vi "Delimited path to array.vi"(8 "error in (no error)":errorcluster, 10 "Node Path Delimited (parent, child)":string, 11 "Tree Map Handle In":T1) -> (0 "error out":errorcluster, 2 "Node Path (parent, child)":string[](array[string]), 3 "Tree Map Handle out":T1)   [LabVIEW 2020, in "Blue Tree Map OpenSource.lvlib"]
doc: "This functions converts a delimited string to a string array.\n\nThis function is particularly useful for converting the delimited string from a LabVIEW tree control to a valid tree path array input for the TreeMap library"
uses:
  Blue Tree Map OpenSource.lvlib
  Typedefs/Tree Map Handle.ctl
  Typedefs/Tree Map.ctl
  Typedefs/Tree Map Data.ctl
  Typedefs/Tree Node Data.ctl
  Typedefs/Attribute Map.ctl
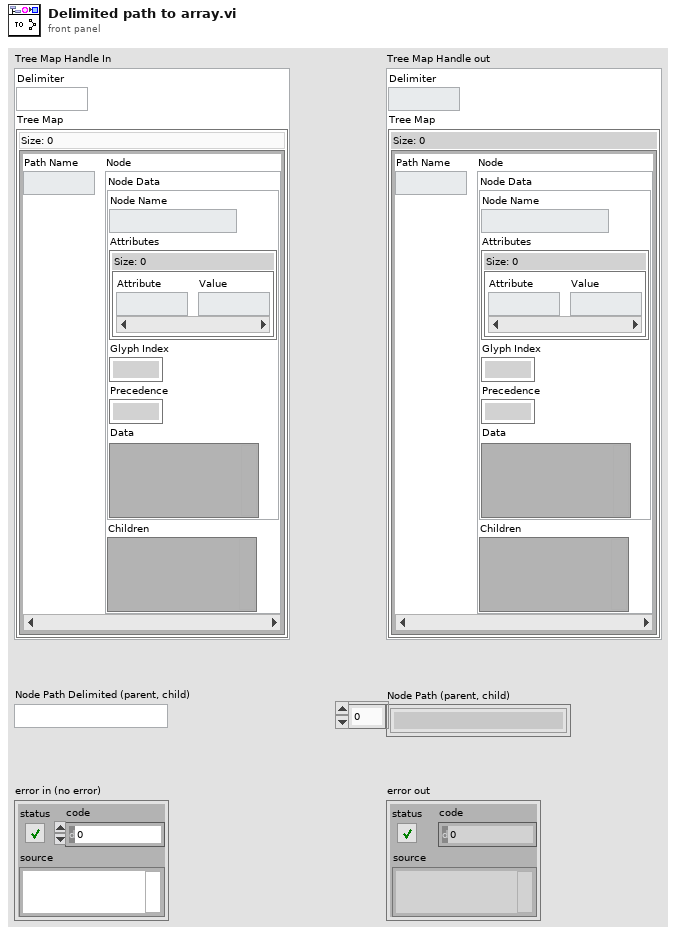
[diagram p1: front panel]
types:
  T1 = typedef "Blue Tree Map OpenSource.lvlib/Tree Map Handle.ctl" = cluster{"Delimiter":string, "Tree Map":T2}
  T2 = typedef "Blue Tree Map OpenSource.lvlib/Tree Map.ctl" = map{string, T3}
  T3 = typedef "Blue Tree Map OpenSource.lvlib/Tree Map Data.ctl" = cluster{"Node Data":T4, "Children":variant}
  T4 = typedef "Blue Tree Map OpenSource.lvlib/Tree Node Data.ctl" = cluster{"Node Name":string, "Attributes":T5, "Glyph Index":i32, "Precedence":i32, "Data":variant}
  T5 = typedef "Blue Tree Map OpenSource.lvlib/Attribute Map.ctl" = map{string, string}
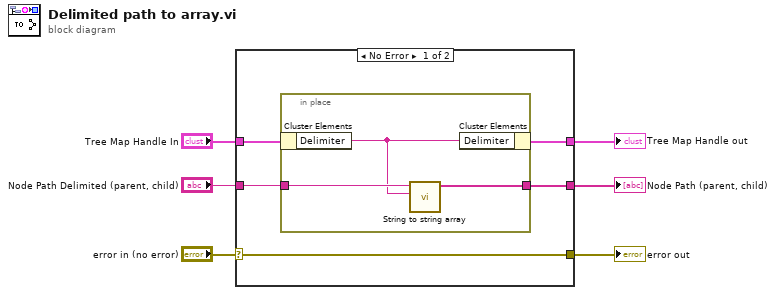
[diagram p0: block diagram]
diagram:
  n1 = case shown="No Error" "error in (no error)" {
    selector: "error in (no error)" -> [w7 w16]
    tunnel: "Tree Map Handle In" -> [w11 w15]
    tunnel: [w10 w15] -> w5
    tunnel: [w7 w16] -> w3
    tunnel: "Node Path Delimited (parent, child)" -> [w9 _]
    tunnel: [w8 _] -> w1
    frame No Error {
      n2 = in-place {
        in-place-border: w9 -> [w14]
        in-place-border: [w12] -> w8
        n3 = in-place-cluster #1(w11) -> ("Delimiter"=w13:string)
        n4 = call "String to string array.vi"("delimiter (\\)"=w13, "String"=w14) -> ("Array"=w12:string[])  [unwired: 9 in]
        n5 = in-place-cluster #1("Delimiter"=w13) -> (w10:T1)
      }
    }
    frame Error {
    }
  }
  "error out" <- w3
  "Tree Map Handle out" <- w5
  "Node Path (parent, child)" <- w1
